vi "Byte47_60 (SubVI).vi"(4 "Card Number":dbl, 5 "Input String":string) -> (0 "Switching Card \nFirmware Version":T1, 1 "Control Card \nConfiguration Version":T2 {"Major Version" format="%.0x"; "Minor Version" format="%.0x"}, 2 "Control Card \nFirmware Version":T1)   [LabVIEW 2024]
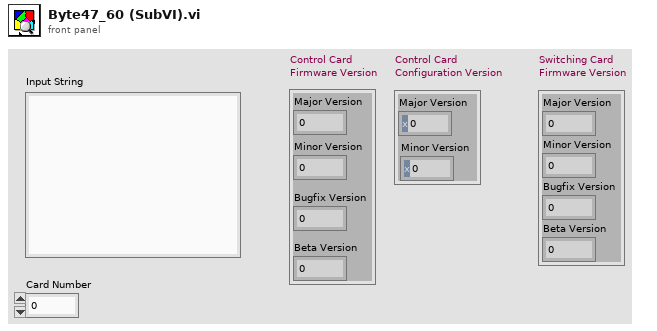
[diagram p1: front panel]
types:
  T1 = cluster{"Major Version":u16, "Minor Version":u16, "Bugfix Version":u16, "Beta Version":u16}
  T2 = cluster{"Minor Version":u16, "Major Version":u16}
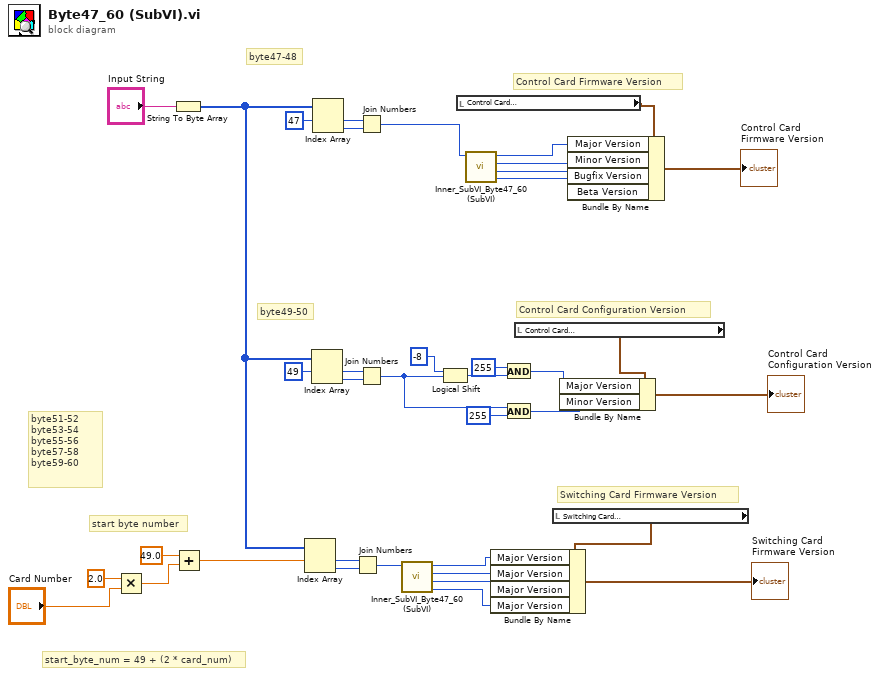
[diagram p0: block diagram]
diagram:
  # "start_byte_num = 49 + (2 * card_num)"
  # "byte51-52\nbyte53-54\nbyte55-56\nbyte57-58\nbyte59-60"
  # "Switching Card Firmware Version"
  # "start byte number"
  # "byte49-50"
  # "Control Card Configuration Version"
  # "Control Card Firmware Version"
  # "byte47-48"
  n1 = Multiply(x=2.0, y="Card Number") -> (x*y=w23:dbl)
  n2 = String To Byte Array(string="Input String") -> (unsigned byte array=w22:u8[])
  n3 = Add(x=49.0, y=w23) -> (x+y=w21:dbl)
  n4 = Index Array "Index Array"(array=w22, index #1=w21) -> (element #1=w19:u8, element #2=w20:u8)  [unwired: 1 in]
  n5 = Index Array "Index Array"(array=w22, index #1=49 ("index")) -> (element #1=w33:u8, element #2=w32:u8)  [unwired: 1 in]
  n6 = Index Array "Index Array"(array=w22, index #1=47 ("index")) -> (element #1=w36:u8, element #2=w35:u8)  [unwired: 1 in]
  n7 = Join Numbers(hi=w19, lo=w20) -> ((hi.lo)=w18:u16)
  n8 = Join Numbers(hi=w36, lo=w35) -> ((hi.lo)=w31:u16)
  n9 = Join Numbers(hi=w33, lo=w32) -> ((hi.lo)=w26:u16)
  n10 = call "Inner_SubVI_Byte47_60 (SubVI).vi"("Numeric in"=w18) -> ("Beta Version"=w7:u16, "Bugfix Version"=w8:u16, "Minor Version"=w9:u16, "Major Version"=w10:u16)  [unwired: 3 in]
  n11 = Logical Shift(y=i16 -8, x=w26) -> (x << y=w28:u16)
  n12 = local read "Control Card \nFirmware Version"() -> (w5:T1)
  n13 = call "Inner_SubVI_Byte47_60 (SubVI).vi"("Numeric in"=w31) -> ("Beta Version"=w13:u16, "Bugfix Version"=w14:u16, "Minor Version"=w15:u16, "Major Version"=w16:u16)  [unwired: 3 in]
  n14 = And(x=u16 255, y=w28) -> (x .and. y?=w12:u16)
  n15 = And(x=w26, y=u16 255) -> (x .and. y?=w11:u16)
  n16 = local read "Control Card \nConfiguration Version"() -> (w3:T2)
  n17 = local read "Switching Card \nFirmware Version"() -> (w2:T1)
  n18 = Bundle By Name(cluster=w2, "Major Version"=w10, "Major Version"=w9, "Major Version"=w8, "Major Version"=w7) -> (→"Switching Card \nFirmware Version":T1)
  n19 = Bundle By Name(cluster=w3, "Major Version"=w12, "Minor Version"=w11) -> (→"Control Card \nConfiguration Version":T2)
  n20 = Bundle By Name(cluster=w5, "Major Version"=w16, "Minor Version"=w15, "Bugfix Version"=w14, "Beta Version"=w13) -> (→"Control Card \nFirmware Version":T1)
